vi "Constructor_RQMHStartup.vi"(7 "Autoshutdown? (T)":bool, 8 "error in (no error)":errorcluster, 10 "StartupParams":variant, 11 "Already Running?":bool) -> (0 "error out":errorcluster, 3 "JQMHStartup out":refnum<class "ModuleStartup.lvclass">)   [LabVIEW 2024, in "ModuleStartup.lvclass"]
uses:
  ModuleStartup.lvclass
  Shared/Died.ctl
  Message.ctl
  Command.ctl
  ModuleStartup.lvclass/ModuleStartup.ctl
  Shared/ModuleShared.lvlib
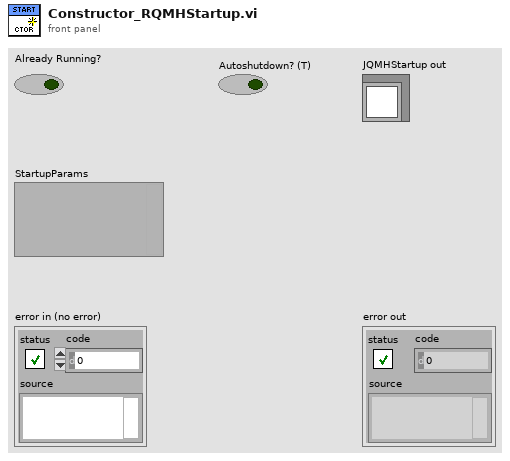
[diagram p1: front panel]
types:
  T1 = typedef "ModuleStartup.lvclass/Message.ctl" = cluster{"Command":T2, "Data":variant}
  T2 = typedef "ModuleStartup.lvclass/Command.ctl" = enum16{"Default", "No Override", "Error", "ACK Created", "ACK Mod Reg", "ACK Caller Reg"}
  T3 = typedef "ModuleShared.lvlib/Died.ctl" = bool
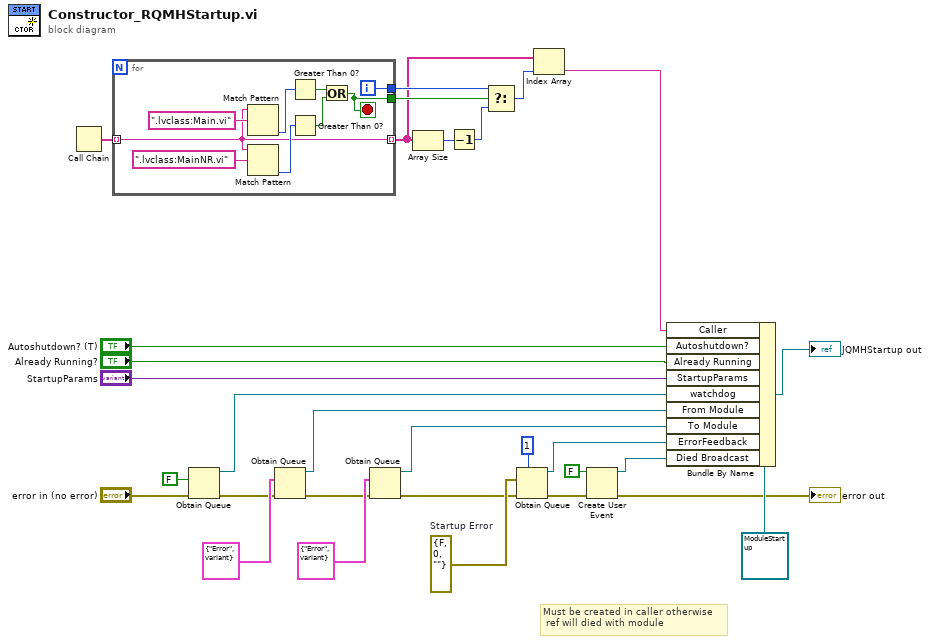
[diagram p0: block diagram]
diagram:
  w20 = errorcluster {"status"=FALSE, "code"=0, "source"=""}  # Startup Error
  # "Must be created in caller otherwise\n ref will died with module"
  n1 = Call Chain() -> (call chain=w10:string[])
  n2 = for {
    tunnel: w10 -> [w33] mode=indexing
    tunnel: [w33] -> w5 mode=indexing
    tunnel: [w32] -> w8
    tunnel: [w31] -> w9
    i -> [w32]
    stop <- w31 stop-if-true
    n3 = Match Pattern(string=w33, regular expression=".lvclass:Main.vi") -> (offset past match=w38:i32)  [unwired: 1 in, 3 out]
    n4 = Match Pattern(string=w33, regular expression=".lvclass:MainNR.vi") -> (offset past match=w37:i32)  [unwired: 1 in, 3 out]
    n5 = Greater Than 0?(x=w38) -> (x > 0?=w35:bool)
    n6 = Greater Than 0?(x=w37) -> (x > 0?=w34:bool)
    n7 = Or(x=w35, y=w34) -> (x .or. y?=w31:bool)
  }
  n8 = Obtain Queue(element data type=FALSE, error in (no error)="error in (no error)") -> (queue out=w16:refnum<queue>, error out=w25:errorcluster)  [unwired: 3 in, 1 out]
  n9 = Obtain Queue(element data type=T1 {"Command"=enum."Error", "Data"=variant} ("Handshake"), error in (no error)=w25) -> (queue out=w17:refnum<queue>, error out=w14:errorcluster)  [unwired: 3 in, 1 out]
  n10 = Obtain Queue(element data type=T1 {"Command"=enum."Error", "Data"=variant} ("Handshake"), error in (no error)=w14) -> (queue out=w12:refnum<queue>, error out=w13:errorcluster)  [unwired: 3 in, 1 out]
  n11 = Array Size(array=w5) -> (size(s)=w7:i32)
  n12 = Decrement(x=w7) -> (x-1=w6:i32)
  n13 = Select(t=w8, s=w9, f=w6) -> (s? t:f=w4:i32)
  n14 = Obtain Queue(max queue size (-1, unlimited)=1, element data type=w20, error in (no error)=w13) -> (queue out=w19:refnum<queue>, error out=w21:errorcluster)  [unwired: 2 in, 1 out]
  n15 = Index Array(array=w5, index=w4) -> (element=w3:string)
  n16 = Create User Event(user event datatype=T3 FALSE ("Died"), error in=w21) -> (user event=w24:refnum<user-event>, error out=→"error out":errorcluster)
  n17 = Bundle By Name(cluster=refnum<class "ModuleStartup.lvclass"> refnum ("JQMHStartup in"), "Caller"=w3, "Autoshutdown?"="Autoshutdown? (T)", "Already Running"="Already Running?", "StartupParams"="StartupParams", "watchdog"=w16, "From Module"=w17, "To Module"=w12, "ErrorFeedback"=w19, "Died Broadcast"=w24) -> (→"JQMHStartup out":refnum<class "ModuleStartup.lvclass">)
